vi "get_IMAQ_ref.vi"(8 "error in (no error)":errorcluster, 11 "Image.lvclass in":refnum<class "Image.lvclass">) -> (0 "error out":errorcluster, 2 "Image":T1, 3 "Image.lvclass out":refnum<class "Image.lvclass">, 4 "not empty?":bool, 6 "empty?":bool)   [LabVIEW 2010, in "Image.lvclass"]
uses:
  Image.lvclass
  <vilib>/vision/Image Controls.llb/IMAQ Image.ctl
  Image.lvclass/Image.ctl
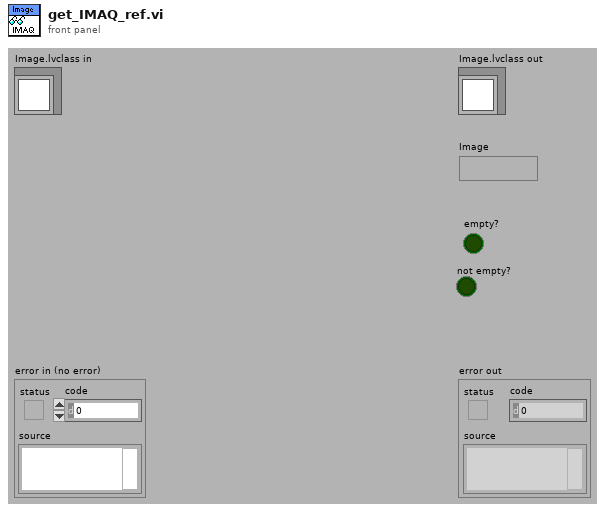
[diagram p1: front panel]
types:
  T1 = typedef "IMAQ Image.ctl" = refnum<image>
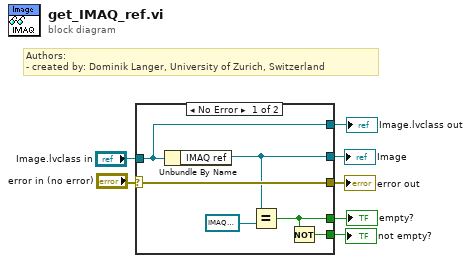
[diagram p0: block diagram]
diagram:
  # "Authors: \n- created by: Dominik Langer, University of Zurich, Switzerland"
  n1 = case shown="No Error" "error in (no error)" {
    selector: "error in (no error)" -> [w12 w14]
    tunnel: [w12 w14] -> w6
    tunnel: [w13 w15] -> w4
    tunnel: "Image.lvclass in" -> [w13 w15]
    tunnel: [w11 _] -> w3
    tunnel: [w9 _] -> w2
    tunnel: [w8 _] -> w1
    frame No Error {
      n2 = Unbundle By Name(w13) -> ("IMAQ ref"=w11:T1)
      n3 = Equal?(x=w11, y=T1 refnum) -> (x = y?=w9:bool)
      n4 = Not(x=w9) -> (.not. x?=w8:bool)
    }
    frame Error {
    }
  }
  "error out" <- w6
  "Image.lvclass out" <- w4
  "Image" <- w3
  "empty?" <- w2
  "not empty?" <- w1
